vi "SMC_SetZero.vi"(8 "error in (no error)":errorcluster) -> (0 "error out":errorcluster)   [LabVIEW 2015]
uses:
  SMC_SubVIs.llb/SMC_ManagerMode.ctl
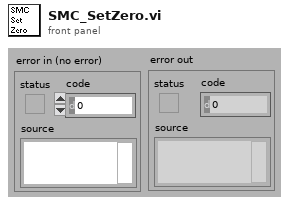
[diagram p1: front panel]
types:
  T1 = typedef "SMC_ManagerMode.ctl" = enum16{"Init", "Get", "SetPosition", "SetStatus", "SetMoving", "SetControllerNr"}
  T2 = typedef "SMC Paras.ctl" = cluster{"VENUS Language":T3, "Number of Axis":u8, "Controller Nr":u8, "Simulation":bool}
  T3 = typedef "VENUSNr.ctl" = enum16{"VENUS 2", "VENUS 1"}
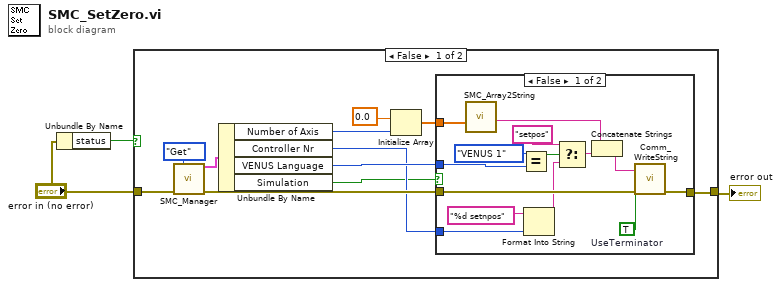
[diagram p0: block diagram]
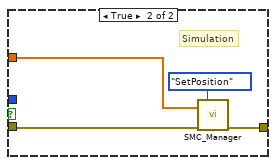
[diagram p2: hidden frame]
diagram:
  n1 = Unbundle By Name("error in (no error)") -> ("status"=w2:bool)
  n2 = case shown="False" w2 {
    tunnel: "error in (no error)" -> [w13 w33]
    tunnel: [w11 w33] -> w1
    frame False {
      n3 = call "SMC_Manager.vi"("Mode"=SMC_ManagerMode."Get", "error in (no error)"=w13) -> ("SMC Parameter Out"=w8:T2, "error out"=w12:errorcluster)  [unwired: 9 in, 3 out]
      n4 = Unbundle By Name(w8) -> ("Number of Axis"=w5:u8, "Controller Nr"=w6:u8, "VENUS Language"=w7:T3, "Simulation"=w4:bool)
      n5 = Initialize Array(0.0, w5) -> (w9:dbl[])
      n6 = case shown="False" w4 {
        tunnel: w12 -> [w28 w31]
        tunnel: [w27 w30] -> w11
        tunnel: w9 -> [w25 w29]
        tunnel: w7 -> [w23 _]
        tunnel: w6 -> [w16 _]
        frame False {
          w15 = TRUE  # UseTerminator
          n7 = call "SMC_Array2String.vi"("Input Array"=w25) -> ("String"=w24:string)  [unwired: 10 in]
          n8 = Equal?(x=enum16{"VENUS 2", "VENUS 1"}."VENUS 1" ("y"), y=w23) -> (x = y?=w21:bool)
          n9 = Format Into String(format string="%d setnpos" ("Format String"), w16) -> (resulting string=w18:string)  [unwired: 2 in, 1 out]
          n10 = Select(t="setpos" ("Substring"), s=w21, f=w18) -> (s? t:f=w19:string)
          n11 = Concatenate Strings(w24, w19) -> (w26:string)
          n12 = call "Comm_WriteString.vi"("string to write"=w26, "error in (no error)"=w28, "UseTerminator"=w15) -> ("error out"=w27:errorcluster)  [unwired: 8 in]
        }
        frame True {
          # "Simulation"
          n13 = call "SMC_Manager.vi"("Mode"=SMC_ManagerMode."SetPosition", "PosArraySimu"=w29, "error in (no error)"=w31) -> ("error out"=w30:errorcluster)  [unwired: 8 in, 4 out]
        }
      }
    }
    frame True {
      # "Error, do nothing"
    }
  }
  "error out" <- w1
